vi "DataVIS_Load some to Intensity DVRy.vi"(8 "error in (no error)":errorcluster, 10 "size to edit":i32, 11 "2D Intensity DVR IN":refnum<data-value>) -> (0 "error out":errorcluster, 3 "2D Intensity DVR OUT":refnum<data-value>)   [LabVIEW 2016]
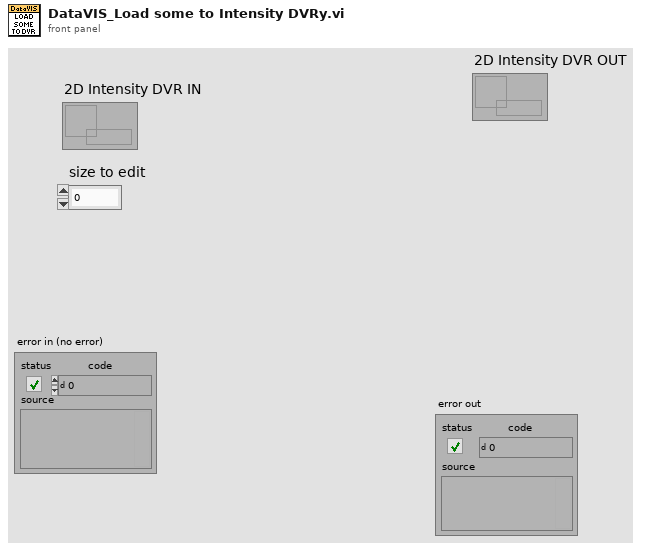
[diagram p1: front panel]
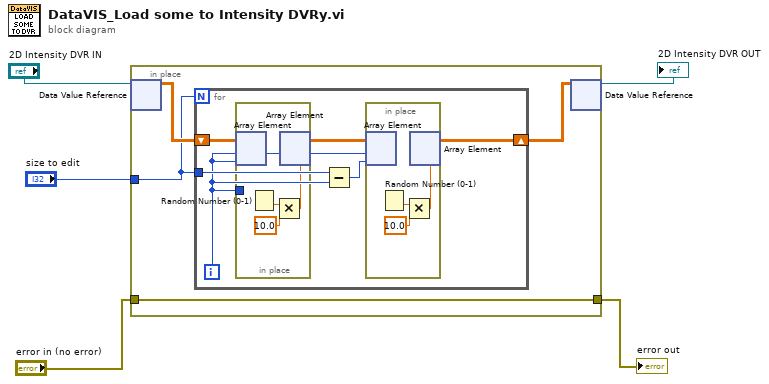
[diagram p0: block diagram]
diagram:
  n1 = in-place {
    in-place-border: "error in (no error)" -> [w9]
    in-place-border: [w9] -> w2
    in-place-border: "size to edit" -> [w6]
    n2 = in-place-dvr #1("2D Intensity DVR IN") -> (w8:dbl[][])  [unwired: 1 out]
    n3 = for {
      N: w6 -> [_]
      shift-right: [w13] -> w7
      shift-left: w8 -> [w15]
      tunnel: w6 -> [w12]
      i -> [w10]
      n4 = in-place {
        in-place-border: w10 -> [_]
        n5 = in-place-array #2(w15, w10, w10) -> ()  [unwired: 1 out]
        n6 = Random Number (0-1)() -> (number: 0 to 1=w21:dbl)
        n7 = Multiply(x=w21, y=10.0) -> (x*y=w19:dbl)
        n8 = in-place-array #2(w19) -> (w14:dbl[][])  [unwired: 2 out]
      }
      n9 = Subtract(x=w12, y=w10) -> (x-y=w11:i32)
      n10 = in-place {
        n11 = in-place-array #3(w14, w10, w11) -> ()  [unwired: 1 out]
        n12 = Random Number (0-1)() -> (number: 0 to 1=w18:dbl)
        n13 = Multiply(x=w18, y=10.0) -> (x*y=w16:dbl)
        n14 = in-place-array #3(w16) -> (w13:dbl[][])  [unwired: 2 out]
      }
    }
    n15 = in-place-dvr #1(w7) -> (→"2D Intensity DVR OUT":refnum<data-value>)  [unwired: 1 out]
  }
  "error out" <- w2
